vi "BuildMsg.vi"(8 "error in (no error)":errorcluster, 10 "Msg to be build":string, 11 "CS++MessageMakerMain in":refnum<class "CS++MessageMakerMain.lvclass">) -> (0 "error out":errorcluster, 3 "CS++MessageMakerMain out":refnum<class "CS++MessageMakerMain.lvclass">)   [LabVIEW 2014, in "CS++MessageMakerMain.lvlib" / "CS++MessageMakerMain.lvclass"]
doc: "Passes the Build Message Command to the specific Actor Instance."
uses:
  CS++MessageMakerMain.lvclass
  CS++MessageMakerMain.lvclass/CS++MessageMakerMain.ctl
  CSPP_Actor/CS++Actor.lvclass/CS++Actor.ctl
  CSPP_Actor/CS++Actor.lvclass
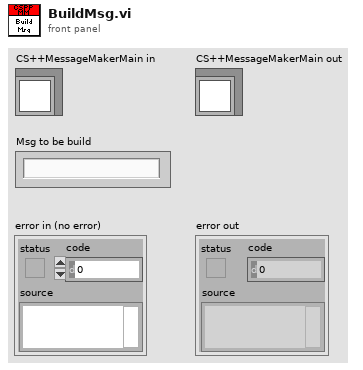
[diagram p1: front panel]
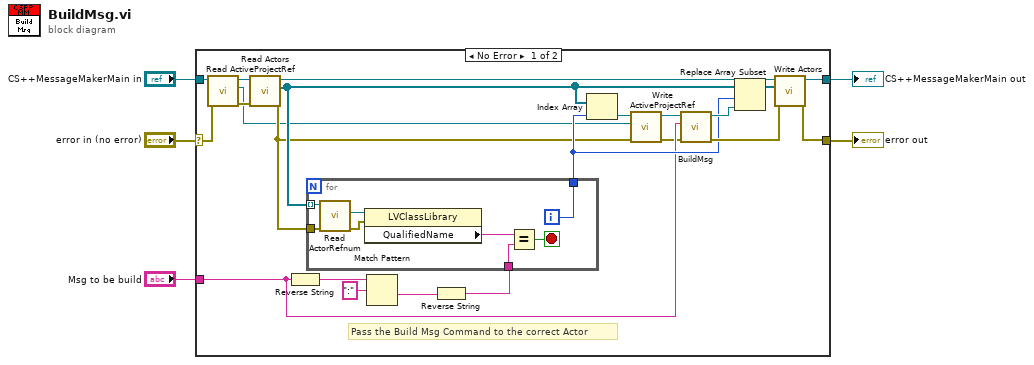
[diagram p0: block diagram]
diagram:
  n1 = case shown="No Error" "error in (no error)" {
    selector: "error in (no error)" -> [w7 w37]
    tunnel: [w25 w37] -> w4
    tunnel: [w24 w36] -> w2
    tunnel: "CS++MessageMakerMain in" -> [w9 w36]
    tunnel: "Msg to be build" -> [w15 _]
    frame No Error {
      # "Pass the Build Msg Command to the correct Actor"
      n2 = call "Read ActiveProjectRef.vi"("error in (no error)"=w7, "CS++MessageMakerMain in"=w9) -> ("error out"=w8:errorcluster, "ActiveProjectRef"=w6:refnum<vi>, "CS++MessageMakerMain out"=w10:refnum<class "CS++MessageMakerMain.lvclass">)  [unwired: 7 in]
      n3 = call "Read Actors.vi"("error in (no error)"=w8, "CS++MessageMakerMain in"=w10) -> ("error out"=w11:errorcluster, "Actors"=w21:refnum<class "CS++Actor.lvclass">[], "CS++MessageMakerMain out"=w27:refnum<class "CS++MessageMakerMain.lvclass">)  [unwired: 7 in]
      n4 = Reverse String(1:w15) -> (0:w20:string)
      n5 = Match Pattern(string=w20, regular expression=":") -> (after substring=w18:string)  [unwired: 1 in, 3 out]
      n6 = Reverse String(1:w18) -> (0:w17:string)
      n7 = for {
        tunnel: w21 -> [w35] mode=indexing
        tunnel: w11 -> [w34]
        tunnel: w17 -> [w30]
        tunnel: [w28] -> w19
        i -> [w28]
        stop <- w29 stop-if-true
        n8 = call "Read ActorRefnum.vi"("error in (no error)"=w34, "CS++Actor in"=w35) -> ("error out"=w32:errorcluster, "ActorRefnum"=w33:refnum<vi>)  [unwired: 7 in, 1 out]
        n9 = property class="LVClassLibrary"(reference=w33, error in=w32) -> ("QualifiedName"=w31:string)  [unwired: 2 out]
        n10 = Equal?(x=w31, y=w30) -> (x = y?=w29:bool)
      }
      n11 = Index Array(array=w21, index=w19) -> (element=w13:refnum<class "CS++Actor.lvclass">)
      n12 = call "Write ActiveProjectRef.vi"("error in (no error)"=w11, "ActiveProjectRef"=w6, "CS++Actor in"=w13) -> ("error out"=w12:errorcluster, "CS++Actor out"=w14:refnum<class "CS++Actor.lvclass">)  [unwired: 7 in]
      n13 = call "BuildMsg.vi"("error in (no error)"=w12, "Msg to be build"=w15, "CS++Actor in"=w14) -> ("error out"=w26:errorcluster, "CS++Actor out"=w22:refnum<class "CS++Actor.lvclass">)  [unwired: 7 in]
      n14 = Replace Array Subset(array=w21, new element=w22, index=w19) -> (w23:refnum<class "CS++Actor.lvclass">[])
      n15 = call "Write Actors.vi"("error in (no error)"=w26, "Actors"=w23, "CS++MessageMakerMain in"=w27) -> ("error out"=w25:errorcluster, "CS++MessageMakerMain out"=w24:refnum<class "CS++MessageMakerMain.lvclass">)  [unwired: 7 in]
    }
    frame Error {
    }
  }
  "error out" <- w4
  "CS++MessageMakerMain out" <- w2
